vi "Err_Code.vi"(8 "错误输入（无错误）":errorcluster caption="Error In(No Error)", 11 "CAN Device In":T1={"Device Type"=20, "Device Index"=0, "CANInd"=0, "Baud(E_U)"=1835016} {"Baud(E_U)" items=["1000Kbps"=393219, "800Kbps"=393220, "500Kbps"=393223, "250Kbps"=1835016, "125Kbps"=1835025, "100Kbps"=1441827, "50Kbps"=1835052, "20Kbps"=1441971, "10Kbps"=1835232, "5Kbps"=1835457]; "Device Type" items=["PCI5121"=1, "PCI9810"=2, "USBCAN1"=3, "USBCAN2"=4, "PCI9820"=5, "PCI5110"=7, "PC104CAN"=11, "CANETUDP"=12, "PCI9840B"=14, "PC104C2"=15, "PCI9820I"=16, "CANETTCP"=17, "PCIE9221"=24, "PCI5010U"=19, "USBCAN_E_U"=20, "USBCAN_2E_U"=21, "PCI5020U"=22, "PCIE9120I"=27, "PCIE9110I"=28, "PCIE9140I"=29, "USBCAN-4E-U"=31, "USBCAN-8E-U"=34]}) -> (0 "错误输出":errorcluster caption="Error Out", 2 "VCI_ERR_INFO":T2, 3 "CAN Device Out":T1={"Device Type"=20, "Device Index"=0, "CANInd"=0, "Baud(E_U)"=1835016} {"Baud(E_U)" items=["1000Kbps"=393219, "800Kbps"=393220, "500Kbps"=393223, "250Kbps"=1835016, "125Kbps"=1835025, "100Kbps"=1441827, "50Kbps"=1835052, "20Kbps"=1441971, "10Kbps"=1835232, "5Kbps"=1835457]; "Device Type" items=["PCI5121"=1, "PCI9810"=2, "USBCAN1"=3, "USBCAN2"=4, "PCI9820"=5, "PCI5110"=7, "PC104CAN"=11, "CANETUDP"=12, "PCI9840B"=14, "PC104C2"=15, "PCI9820I"=16, "CANETTCP"=17, "PCIE9221"=24, "PCI5010U"=19, "USBCAN_E_U"=20, "USBCAN_2E_U"=21, "PCI5020U"=22, "PCIE9120I"=27, "PCIE9110I"=28, "PCIE9140I"=29, "USBCAN-4E-U"=31, "USBCAN-8E-U"=34]})   [LabVIEW 2020, in "ZLGCAN.lvclass"]
uses:
  ZLGCAN.lvclass
  Device.ctl
  ControlCAN.dll
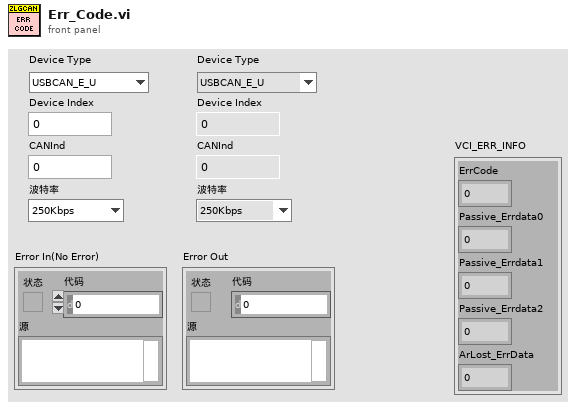
[diagram p1: front panel]
types:
  T1 = typedef "ZLGCAN.lvclass/Device.ctl" = cluster{"Device Type":u32, "Device Index":u32, "CANInd":u32, "Baud(E_U)":u32}
  T2 = cluster{"ErrCode":u32, "Passive_Errdata0":u8, "Passive_Errdata1":u8, "Passive_Errdata2":u8, "ArLost_ErrData":u32}
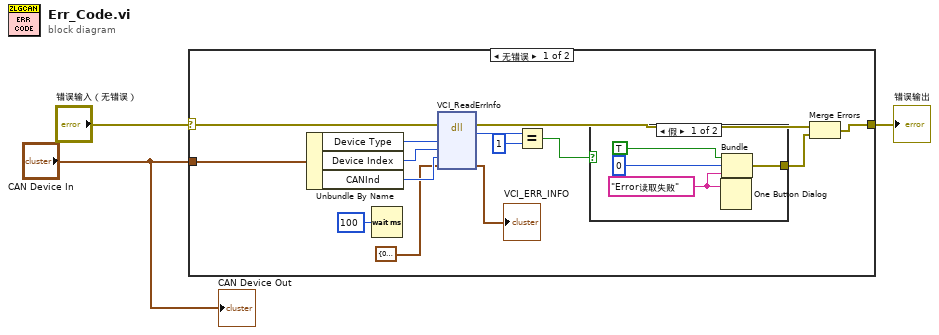
[diagram p0: block diagram]
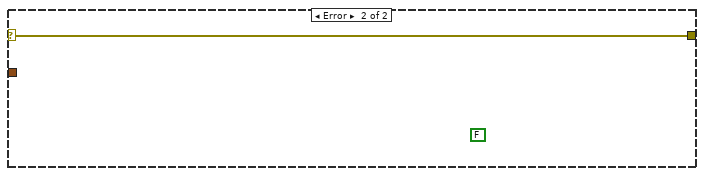
[diagram p3: hidden frame]
diagram:
  n1 = case shown="无错误" "错误输入（无错误）" {
    selector: "错误输入（无错误）" -> [w7 w22]
    tunnel: [w14 w22] -> w2
    tunnel: "CAN Device In" -> [w6 _]
    frame No Error {
      n2 = Unbundle By Name(w6) -> ("Device Type"=w11:u32, "Device Index"=w10:u32, "CANInd"=w9:u32)
      n3 = Wait (ms)(milliseconds to wait=u32 100 ("等待时间（毫秒）")) -> ()  [unwired: 1 out]
      n4 = dll-call lib="PTH2sabs CUsersxu.dongDesktop新建文件夹新建文件夹 (2) - 副本ZLGCAN\nControlCANControlCAN.dll" fn="VCI_ReadErrInfo"(error in=w7, "DeviceType"=w11, "DeviceInd"=w10, "CANInd"=w9, "PErrInfo"=T2 {"ErrCode"=0, "Passive_Errdata0"=0, "Passive_Errdata1"=0, "Passive_Errdata2"=0, "ArLost_ErrData"=0} ("VCI_ERR_INFO")) -> (error out=w13:errorcluster, "返回类型"=w12:u32, "PErrInfo"=→"VCI_ERR_INFO":T2)  [unwired: 5 in, 1 out]
      n5 = Equal?(x=w12, y=u32 1) -> (x = y?=w15:bool)
      n6 = case shown="假" w15 {
        tunnel: [w18 _] -> w16
        frame False {
          w21 = "Error读取失败" ("消息")
          n7 = One Button Dialog(message=w21) -> ()  [unwired: 1 in, 1 out]
          n8 = Bundle("status"=TRUE, "code"=0, "消息"=w21) -> (w18:cluster{"status":bool, "code":i32, "消息":string})  [unwired: 1 in]
        }
        frame True {
        }
      }
      n9 = Merge Errors(w13, w16) -> (w14:errorcluster)
    }
    frame Error {
      (unwired) FALSE
    }
  }
  "错误输出" <- w2
  "CAN Device Out" <- "CAN Device In"
